vi "ReadPreScale.vi"(8 "error in (no error)":errorcluster, 11 "PCA in":refnum<class "PCA.lvclass">) -> (0 "error out":errorcluster, 2 "Prescale":u8, 3 "PCA out":refnum<class "PCA.lvclass">)   [LabVIEW 2022 SP3, in "PCA9685.lvlib" / "PCA.lvclass"]
uses:
  PCA.lvclass
  PCA.lvclass/PCA.ctl
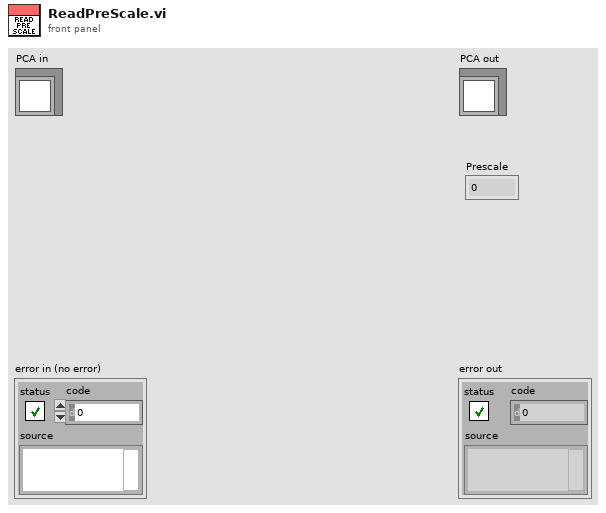
[diagram p1: front panel]
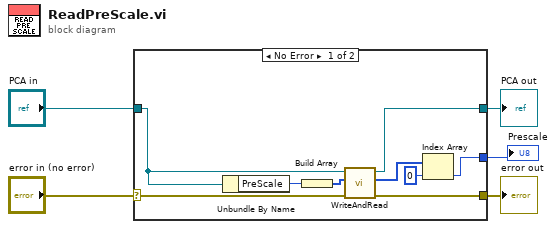
[diagram p0: block diagram]
diagram:
  n1 = case shown="No Error" "error in (no error)" {
    selector: "error in (no error)" -> [w14 w16]
    tunnel: [w13 w16] -> w4
    tunnel: [w12 w15] -> w2
    tunnel: "PCA in" -> [w11 w15]
    tunnel: [w6 _] -> w1
    frame No Error {
      n2 = Unbundle By Name(w11) -> ("PreScale"=w10:u8)
      n3 = Build Array(w10) -> (w9:u8[])
      n4 = call "WriteAndRead.vi"("error in (no error)"=w14, "Data"=w9, "PCA in"=w11) -> ("error out"=w13:errorcluster, "Data 2"=w8:u8[], "PCA out"=w12:refnum<class "PCA.lvclass">)  [unwired: 6 in]
      n5 = Index Array(array=w8, index=0) -> (element=w6:u8)
    }
    frame Error {
    }
  }
  "error out" <- w4
  "PCA out" <- w2
  "Prescale" <- w1
